vi "LoadNodeUIStandardEvents.vi"(7 "user event out":T1, 8 "error in":errorcluster, 9 "sub panel ref in":refnum<vi>, 10 "main queue":T8, 11 "node":T7) -> (0 "error out":errorcluster)   [LabVIEW 2013, in "NISE_CEF_TreeControl.lvlib"]
doc: "This VI will insert the UI from a node into a subpanel."
uses:
  NISE_CEF_TreeControl.lvlib
  <vilib>/NI/AMC/Message Queue.ctl
  <vilib>/NI/AMC/Message.ctl
  <vilib>/NI/Tools/Keyed Array/KeyedArray.ctl
  Node/NodeRef.ctl
  Node/NISE_CEF_Node.lvclass
  Node/StandardEvents.ctl
  Node/UserEventRef.ctl
  Controls/EventCluster.ctl
  Node/NodeChangeEvent.ctl
  Node/CacheState.ctl
  Node/RefreshUIEvent.ctl
  Node/StopEvent.ctl
  <vilib>/NI/Tools/Keyed Array/Tools_KeyedArray.lvlib
  <vilib>/NI/AMC/AMC.lvlib
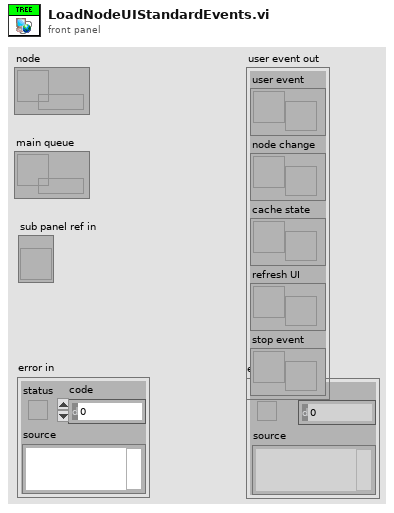
[diagram p1: front panel]
types:
  T1 = typedef "NISE_CEF_Node.lvclass/StandardEvents.ctl" = cluster{"user event":T2, "node change":T3, "cache state":T4, "refresh UI":T5, "stop event":T6}
  T2 = typedef "NISE_CEF_Node.lvclass/UserEventRef.ctl" = refnum<user-event>
  T3 = typedef "NISE_CEF_Node.lvclass/NodeChangeEvent.ctl" = refnum<user-event>
  T4 = typedef "NISE_CEF_Node.lvclass/CacheState.ctl" = refnum<user-event>
  T5 = typedef "NISE_CEF_Node.lvclass/RefreshUIEvent.ctl" = refnum<user-event>
  T6 = typedef "NISE_CEF_Node.lvclass/StopEvent.ctl" = refnum<user-event>
  T7 = typedef "NISE_CEF_Node.lvclass/NodeRef.ctl" = refnum<data-value>
  T8 = typedef "AMC.lvlib/Message Queue.ctl" = refnum<queue>
  T9 = enum32{"Bad", "Idle", "Run top level", "Running"}
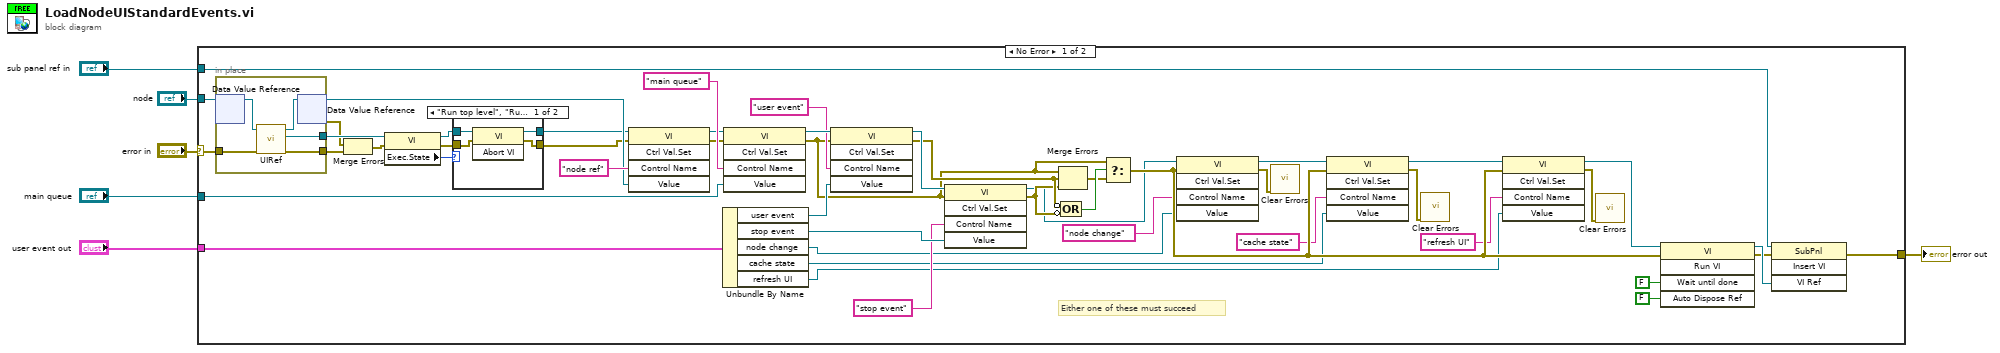
[diagram p0: block diagram]
diagram:
  n1 = case shown="No Error" "error in" {
    selector: "error in" -> [w44 w67]
    tunnel: [w7 w67] -> w5
    tunnel: "node" -> [w37 _]
    tunnel: "main queue" -> [w36 _]
    tunnel: "user event out" -> [w31 _]
    tunnel: "sub panel ref in" -> [w35 _]
    frame No Error {
      # "Either one of these must succeed"
      n2 = in-place {
        in-place-border: w44 -> [w63]
        in-place-border: [w64] -> w43
        in-place-border: [w62] -> w34
        n3 = in-place-dvr #1(w37) -> (w66:refnum<class "NISE_CEF_Node.lvclass">)  [unwired: 1 out]
        n4 = call-dynamic "UIRef.vi"("error in"=w63, "node in"=w66) -> ("error out"=w62:errorcluster, "VI refnum"=w64:refnum<vi>, "node out"=w65:refnum<class "NISE_CEF_Node.lvclass">)  [unwired: 7 in]
        n5 = in-place-dvr #1(w65) -> (w45:T7, w33:errorcluster)
      }
      n6 = Merge Errors(w33, w34) -> (w32:errorcluster)
      n7 = property class="VI"(reference=w43, error in=w32) -> (reference out=w40:refnum<vi>, error out=w39:errorcluster, "Exec.State"=w42:T9)
      n8 = case shown="\"Run top level\", \"Running\"" w42 {
        tunnel: [w56 w61] -> w41
        tunnel: w40 -> [w59 w61]
        tunnel: w39 -> [w58 w60]
        tunnel: [w57 w60] -> w38
        frame "Run top level", "Running" {
          n9 = invoke class="VI" method="Abort VI"(reference=w59, error in=w58) -> (reference out=w56:refnum<vi>, error out=w57:errorcluster)  [unwired: 1 in, 1 out]
        }
        frame "Idle", Default {
        }
      }
      n10 = invoke class="VI" method="Ctrl Val.Set"(reference=w41, error in=w38, "Control Name"="node ref", "Value"=w45) -> (reference out=w53:refnum<vi>, error out=w48:errorcluster)  [unwired: 1 in, 3 out]
      n11 = Unbundle By Name(w31) -> ("user event"=w30:T2, "stop event"=w28:T6, "node change"=w13:T3, "cache state"=w12:T4, "refresh UI"=w11:T5)
      n12 = invoke class="VI" method="Ctrl Val.Set"(reference=w53, error in=w48, "Control Name"="main queue", "Value"=w36) -> (reference out=w47:refnum<vi>, error out=w22:errorcluster)  [unwired: 1 in, 3 out]
      n13 = invoke class="VI" method="Ctrl Val.Set"(reference=w47, error in=w22, "Control Name"="user event", "Value"=w30) -> (reference out=w29:refnum<vi>, error out=w26:errorcluster)  [unwired: 1 in, 3 out]
      n14 = invoke class="VI" method="Ctrl Val.Set"(reference=w29, error in=w22, "Control Name"="stop event", "Value"=w28) -> (reference out=w20:refnum<vi>, error out=w25:errorcluster)  [unwired: 1 in, 3 out]
      n15 = Merge Errors(w22, w26, w25) -> (w23:errorcluster)
      n16 = Compound Arithmetic op=OR(invert w26, invert w25) -> (w24:bool)
      n17 = Select(t=w22, s=w24, f=w23) -> (s? t:f=w21:errorcluster)
      n18 = invoke class="VI" method="Ctrl Val.Set"(reference=w20, error in=w21, "Control Name"="node change", "Value"=w13) -> (reference out=w19:refnum<vi>, error out=w9:errorcluster)  [unwired: 1 in, 3 out]
      n19 = call <vilib>:"Clear Errors.vi"("error in (no error)"=w9) -> ()  [unwired: 6 in, 1 out]
      n20 = invoke class="VI" method="Ctrl Val.Set"(reference=w19, error in=w21, "Control Name"="cache state", "Value"=w12) -> (reference out=w18:refnum<vi>, error out=w10:errorcluster)  [unwired: 1 in, 3 out]
      n21 = call <vilib>:"Clear Errors.vi"("error in (no error)"=w10) -> ()  [unwired: 6 in, 1 out]
      n22 = invoke class="VI" method="Ctrl Val.Set"(reference=w18, error in=w21, "Control Name"="refresh UI", "Value"=w11) -> (reference out=w17:refnum<vi>, error out=w8:errorcluster)  [unwired: 1 in, 3 out]
      n23 = call <vilib>:"Clear Errors.vi"("error in (no error)"=w8) -> ()  [unwired: 6 in, 1 out]
      n24 = invoke class="VI" method="Run VI"(reference=w17, error in=w21, "Wait until done"=FALSE ("Wait Until Done"), "Auto Dispose Ref"=FALSE ("Auto Dispose Reference")) -> (reference out=w52:refnum<vi>, error out=w51:errorcluster)  [unwired: 1 in, 3 out]
      n25 = invoke class="SubPnl" method="Insert VI"(reference=w35, error in=w51, "VI Ref"=w52) -> (error out=w7:errorcluster)  [unwired: 1 in, 3 out]
    }
    frame Error {
    }
  }
  "error out" <- w5
